vi "To Serial Form.vi"(6 "Serial Version":T1, 10 "Serializer in":refnum<class "Serializer.lvclass">, 11 "Alicat in":refnum<class "Alicat.lvclass">) -> (0 "error out":errorcluster, 2 "Serializer out":refnum<class "Serializer.lvclass">, 3 "Alicat out":refnum<class "Alicat.lvclass">)   [LabVIEW 2012]
uses:
  <userlib>/Serialization/Serializable/Serializable.lvclass
  <userlib>/Serialization/Serializable/Insert Boolean.vi
  <userlib>/Serialization/Serializable/Insert Int16.vi
  Controls/Gas.ctl
  Alicat.lvclass
  <userlib>/Serialization/Serializable/Insert String.vi
  <userlib>/Serialization/Serializer/Serializer.lvclass
  <userlib>/Serialization/Serialization Common/Serial Version.ctl
  <userlib>/Serialization/Serialization Common/Serialization Common.lvlib
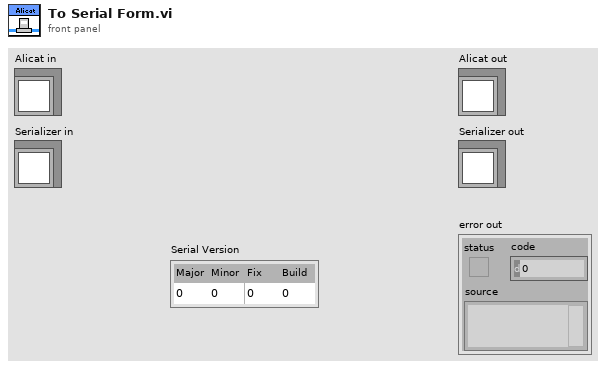
[diagram p1: front panel]
types:
  T1 = typedef "Serialization Common.lvlib/Serial Version.ctl" = cluster{"Major":u16, "Minor":u16, "Fix":u16, "Build":u16}
  T2 = typedef "Alicat.lvlib/Alicat.lvclass/Gas.ctl" = enum16{"Air", "Ar", "CH4", "CO", "CO2", "C2H6", "H2", "He", "N2", "NO", "Ne", "O2", "C3H8", "n-C4H10", "C2H2", "C2H4", "i-C2H10", "Kr", "Xe"}
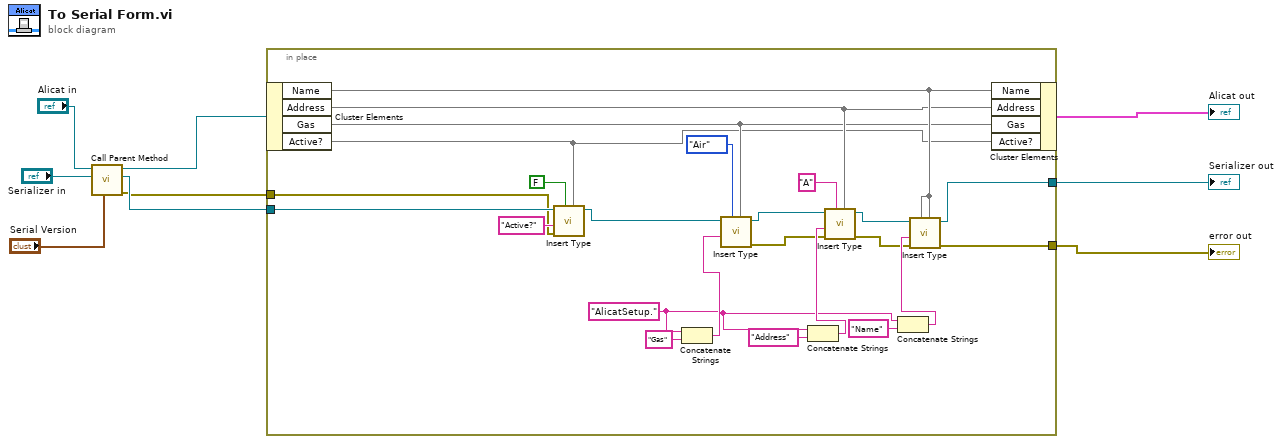
[diagram p0: block diagram]
diagram:
  n1 = call-parent "Call Parent Method"("Serial Version"="Serial Version", "Serializer in"="Serializer in", "Serializable in"="Alicat in") -> ("error out"=w4:errorcluster, "Serializer out"=w5:refnum<class "Serializer.lvclass">, "Serializable out"=w6:refnum<class "Serializable.lvclass">)  [unwired: 6 in]
  n2 = in-place {
    in-place-border: w5 -> [w33]
    in-place-border: w4 -> [w30]
    in-place-border: [w15] -> w3
    in-place-border: [w14] -> w1
    w19 = "AlicatSetup."
    n3 = in-place-cluster #1(w6) -> ("Name"=w13, "Address"=w12, "Gas"=w11, "Active?"=w10)
    n4 = call-poly <userlib>:"Insert Type.vi"("Boolean"=w10, "Default Value"=FALSE, "error in (no error)"=w30, "Name"="Active?", "Serializer in"=w33) -> ("Serializer out"=w27:refnum<class "Serializer.lvclass">)  [unwired: 5 in, 1 out]
    n5 = Concatenate Strings(w19, "Gas" ("string")) -> (w28:string)
    n6 = call-poly <userlib>:"Insert Type.vi"("Integer"=w11, "Default Value"=Gas."Air" ("AlicatSetup.Gas"), "Name"=w28, "Serializer in"=w27) -> ("error out"=w21:errorcluster, "Serializer out"=w24:refnum<class "Serializer.lvclass">)  [unwired: 6 in]
    n7 = Concatenate Strings(w19, "Address" ("string")) -> (w22:string)
    n8 = call-poly <userlib>:"Insert Type.vi"("String"=w12, "Default Value"="A", "error in (no error)"=w21, "Name"=w22, "Serializer in"=w24) -> ("error out"=w16:errorcluster, "Serializer out"=w20:refnum<class "Serializer.lvclass">)  [unwired: 5 in]
    n9 = Concatenate Strings(w19, "Name" ("string")) -> (w17:string)
    n10 = call-poly <userlib>:"Insert Type.vi"("Boolean"=w13, "Default Value"=w13, "error in (no error)"=w16, "Name"=w17, "Serializer in"=w20) -> ("error out"=w14:errorcluster, "Serializer out"=w15:refnum<class "Serializer.lvclass">)  [unwired: 5 in]
    n11 = in-place-cluster #1("Name"=w13, "Address"=w12, "Gas"=w11, "Active?"=w10) -> (→"Alicat out":cluster{})
  }
  "error out" <- w1
  "Serializer out" <- w3
